vi "NIIE_IsAntsRectValid.vi"(11 "Image Range":T1) -> (3 "Valid? Out":bool, 5 "Max. Rect Size? Out":bool)   [LabVIEW 2021]
uses:
  <vilib>/Utility/miscctls.llb/LVRectTypeDef.ctl
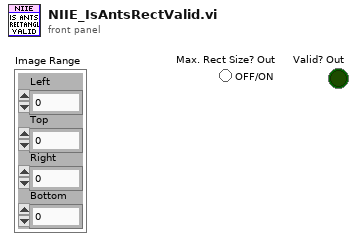
[diagram p1: front panel]
types:
  T1 = typedef "LVRectTypeDef.ctl" = cluster{"Left":i16, "Top":i16, "Right":i16, "Bottom":i16}
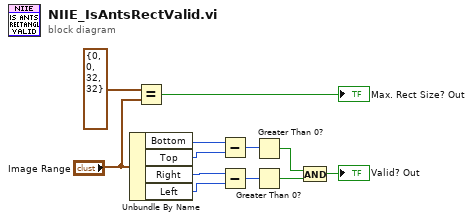
[diagram p0: block diagram]
diagram:
  n1 = Unbundle By Name("Image Range") -> ("Bottom"=w12:i16, "Top"=w11:i16, "Right"=w10:i16, "Left"=w9:i16)
  n2 = Equal?(x=T1 {"Left"=0, "Top"=0, "Right"=32, "Bottom"=32} ("Image Range"), y="Image Range") -> (x = y?=→"Max. Rect Size? Out":bool)
  n3 = Subtract(x=w12, y=w11) -> (x-y=w8:i16)
  n4 = Subtract(x=w10, y=w9) -> (x-y=w7:i16)
  n5 = Greater Than 0?(x=w8) -> (x > 0?=w5:bool)
  n6 = Greater Than 0?(x=w7) -> (x > 0?=w6:bool)
  n7 = And(x=w5, y=w6) -> (x .and. y?=→"Valid? Out":bool)
